vi "LCD_read.vi"() -> ()   [LabVIEW 2017]
doc: "This example shows how to use the NI Vision seven-segment display reader VIs to read values that are displayed on a LCD panel."
uses:
  <vilib>/vision/NI_Vision_Development_Module.lvlib
panel:
  out "Image":T1(plugin-control)
  out "Segments status":T2(array[cluster])
  in  "Delay":i32(slide)=738 max=3000 scale=0.0..1000.0
  out "Output value":dbl
  in  "stop":bool
  # "Overview\nThis is the file for the example mentioned here. As of LabVIEW 2013, this example is no longer installs with the Vision Development Module examples.\n I've posted it here so that users who want the example in later versions of LabVIEW can have access to it..\nRequirements\nLabVIEW and the Vision Development Module 2013 and later (for this file). If you have a version of LabVIEW that is earlier than 2013, the example should\nhave installed on your system with the Vision Development Module\nInstructions\nJust run this VI and observe the Front Panel as the VI inspects the sample images"
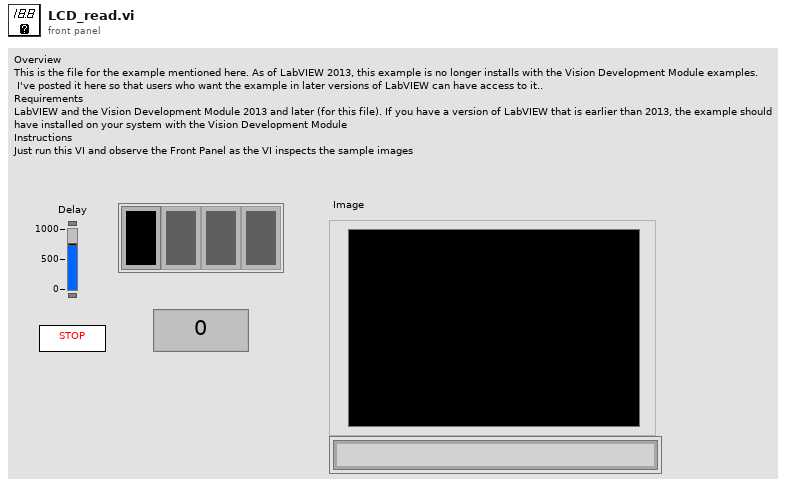
[diagram p1: front panel]
types:
  T1 = typedef "IMAQ Image.ctl" = refnum<image>
  T2 = cluster{bool, bool, bool, bool, bool, bool, bool}[]
  T3 = cluster{i32[], cluster{"Contour Type":u32, "ROI Type":u32, i32[]}[]}
  T4 = cluster{"Global Rectangle":i32[], "Contours":cluster{"ID":enum32{"External", "Internal"}, "Type":u32, "Coordinates":i32[]}[]}
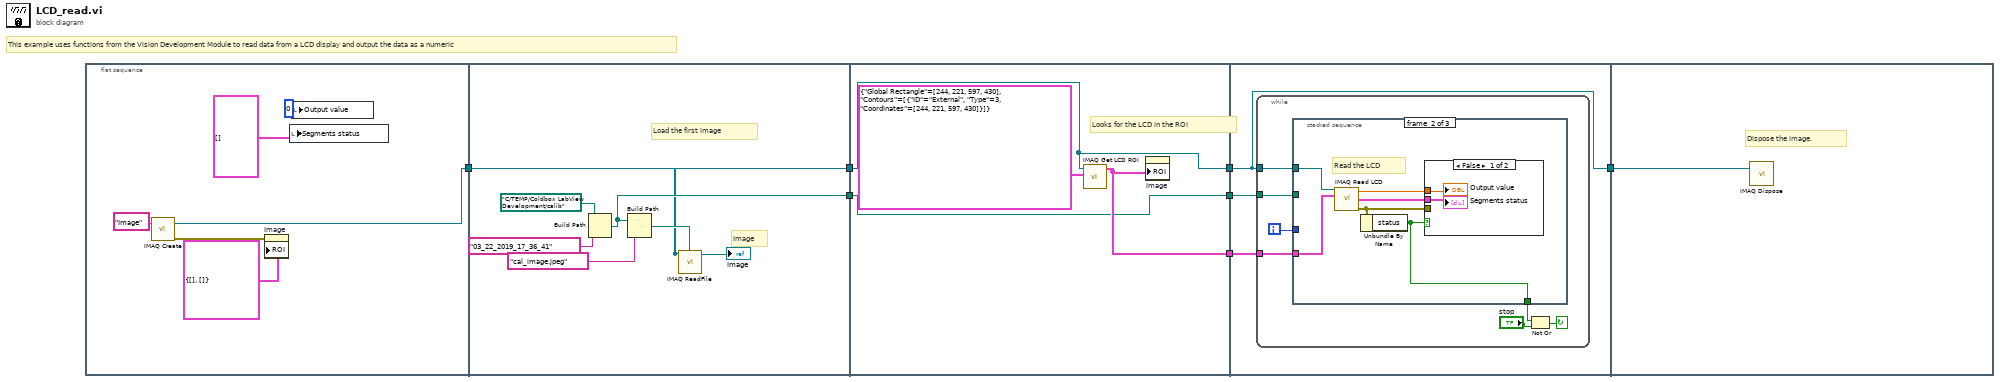
[diagram p0: block diagram]
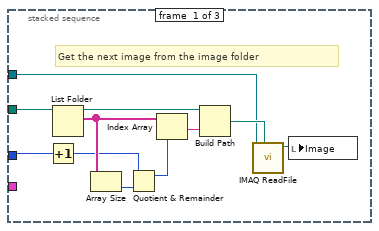
[diagram p2: hidden frame]
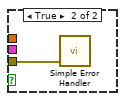
[diagram p3: hidden frame]
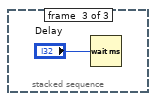
[diagram p4: hidden frame]
diagram:
  # "This example uses functions from the Vision Development Module to read data from a LCD display and output the data as a numeric"
  n1 = flat-sequence {
    tunnel: [w12] -> w7
    tunnel: w7 -> [w16]
    tunnel: [w16] -> w6
    tunnel: [w17] -> w5
    tunnel: w6 -> [w24]
    tunnel: [w24] -> w4
    tunnel: [w23] -> w3
    tunnel: w5 -> [w21]
    tunnel: [w21] -> w2
    tunnel: w4 -> [w26]
    tunnel: [w26] -> w1
    tunnel: w3 -> [w27]
    tunnel: w2 -> [w25]
    tunnel: w1 -> [w56]
    frame #0 {
      n2 = call "IMAQ Create"("Image Name"="Image") -> ("New Image"=w12:T1, "error out"=w9:errorcluster)  [unwired: 3 in, 1 out]
      n3 = property on="Image" class="ImageControl"(error in=w9, "ROI"=T3 {[], []}) -> ()  [unwired: 1 in, 2 out]
      n4 = local write "Segments status"(T2 [] ("Segments status")) -> ()
      n5 = local write "Output value"(0 ("Output value")) -> ()
    }
    frame #1 {
      # "Image"
      # "Load the first image"
      n6 = Build Path(base path=path "C:/TEMP/Coldbox LabView Development/calib", name or relative path="03_22_2019_17_36_41") -> (appended path=w17:path)
      n7 = Build Path(base path=w17, name or relative path="cal_image.jpeg") -> (appended path=w18:path)
      n8 = call "IMAQ ReadFile"("File Path"=w18, "Image"=w16) -> ("Image Out"=→"Image":T1)  [unwired: 3 in, 6 out]
    }
    frame #2 {
      # "Looks for the LCD in the ROI"
      n9 = call "IMAQ Get LCD ROI"("ROI Descriptor"=T4 {"Global Rectangle"=[244, 221, 597, 430], "Contours"=[{"ID"=enum."External", "Type"=3, "Coordinates"=[244, 221, 597, 430]}]}, "Image"=w24) -> ("ROI Descriptor out"=w23:T4)  [unwired: 3 in, 6 out]
      n10 = property on="Image" class="ImageControl"("ROI"=w23) -> ()  [unwired: 2 in, 2 out]
    }
    frame #3 {
      n11 = while {
        tunnel: w25 -> [w29]
        tunnel: w26 -> [w31]
        tunnel: w27 -> [w33]
        i -> [w30]
        stop <- w32 continue-if-true
        n12 = stacked-sequence {
          tunnel: w33 -> [_ w51 _]
          tunnel: w31 -> [w38 w48 _]
          tunnel: w30 -> [w37 _ _]
          tunnel: w29 -> [w36 _ _]
          tunnel: [_ w47 _] -> w28
          frame #0 {
            # "Get the next image from the image folder"
            n13 = Increment(x=w37) -> (x+1=w39:i32)
            n14 = List Folder(path=w36) -> (path out=w41:path, filenames=w45:string[])  [unwired: 1 in, 4 out]
            n15 = Array Size(array=w45) -> (size(s)=w44:i32)
            n16 = Quotient & Remainder(x=w39, y=w44) -> (x-y*floor(x/y)=w43:i32)  [unwired: 1 out]
            n17 = Index Array(array=w45, index=w43) -> (element=w42:string)
            n18 = Build Path(base path=w41, name or relative path=w42) -> (appended path=w40:path)
            n19 = call "IMAQ ReadFile"("File Path"=w40, "Image"=w38) -> ("Image Out"=w35:T1)  [unwired: 3 in, 6 out]
            n20 = local write "Image"(w35) -> ()
          }
          frame #1 {
            # "Read the LCD"
            n21 = call "IMAQ Read LCD"("Image"=w48, "ROI Descriptor"=w51) -> ("Output value"=w50:dbl, "Segments status"=w49:T2, "error out"=w46:errorcluster)  [unwired: 5 in, 6 out]
            n22 = Unbundle By Name(w46) -> ("status"=w47:bool)
            n23 = case shown="False" w47 {
              tunnel: w50 -> [w53 _]
              tunnel: w49 -> [w52 _]
              tunnel: w46 -> [_ w54]
              frame False {
                "Output value" <- w53
                "Segments status" <- w52
              }
              frame True {
                n24 = call <vilib>:"Simple Error Handler.vi"("error in (no error)"=w54) -> ()  [unwired: 1 in, 8 out]
              }
            }
          }
          frame #2 {
            n25 = Wait (ms)(milliseconds to wait="Delay") -> ()  [unwired: 1 out]
          }
        }
        n26 = Not Or(1:"stop", 2:w28) -> (0:w32:bool)
      }
    }
    frame #4 {
      # "Dispose the image."
      n27 = call "IMAQ Dispose"("Image"=w56) -> ()  [unwired: 2 in, 4 out]
    }
  }
